vi "Read Customer Name.vi"(8 "error in (no error)":errorcluster, 11 "Order in":refnum<class "Order.lvclass">) -> (0 "error out":errorcluster, 2 "Customer Name":string, 3 "Order out":refnum<class "Order.lvclass">)   [LabVIEW 2023, in "Order.lvclass"]
doc: "Read Customer Name accessor VI"
uses:
  Order.lvclass
  Order.lvclass/Order.ctl
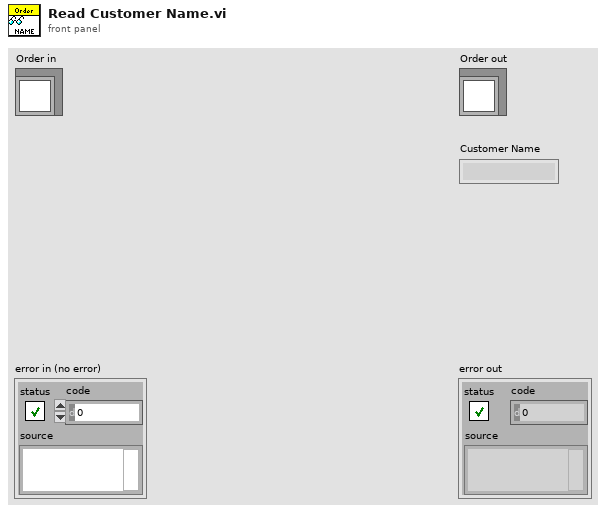
[diagram p1: front panel]
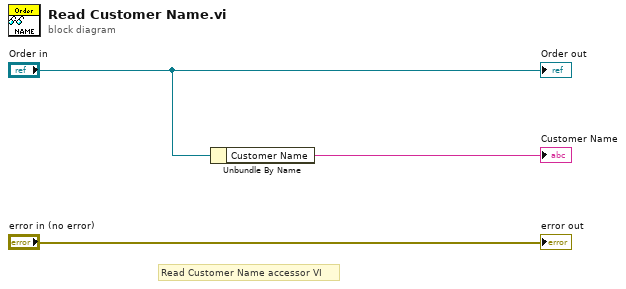
[diagram p0: block diagram]
diagram:
  # "Read Customer Name accessor VI"
  n1 = Unbundle By Name("Order in") -> ("Customer Name"=→"Customer Name":string)
  "error out" <- "error in (no error)"
  "Order out" <- "Order in"
